vi "validate line configuration.vi"(7 "module":refnum<class "Scan Engine configuration.lvclass">, 11 "Mappings in":T1) -> (1 "valid?":bool, 2 "errors":string, 3 "Mappings out":T1)   [LabVIEW 2013, in "Scan Engine editor node.lvclass"]
uses:
  Scan Engine editor node.lvclass
  Mappings.ctl
  <vilib>/NI/Tag Bus Module Framework/channel/TBM channel.lvclass
  module/configuration/Line.ctl
  Map.ctl
  module/configuration/Scan Engine configuration.lvclass
  <vilib>/NI/Tag Bus/tag/tag descriptor.lvclass/tag descriptor.ctl
  <vilib>/NI/Tag Bus/tag/read tag name.vi
panel:
  in  "warn?":bool
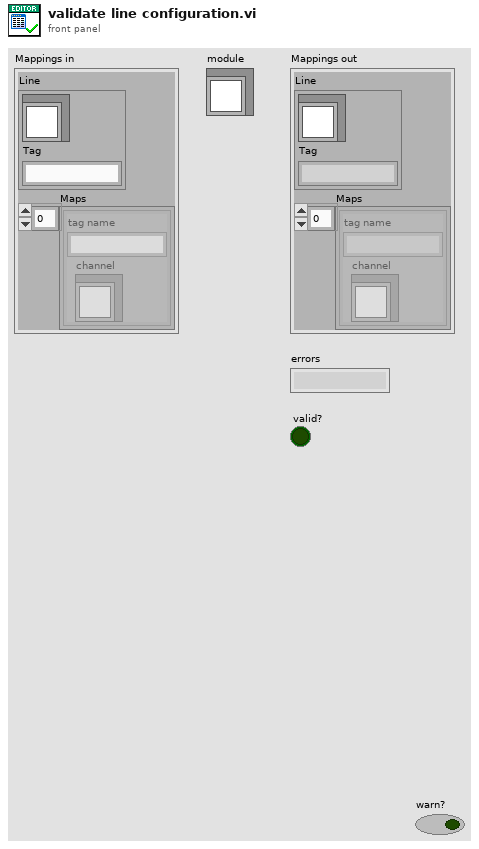
[diagram p1: front panel]
types:
  T1 = typedef "Scan Engine editor node.lvclass/Mappings.ctl" = cluster{"Line":T2, "Maps":T3[]}
  T2 = typedef "Scan Engine configuration.lvclass/Line.ctl" = cluster{"channel":refnum<class "TBM channel.lvclass">, "Tag":string}
  T3 = typedef "Scan Engine editor node.lvclass/Map.ctl" = cluster{"channel":refnum<class "TBM channel.lvclass">, "tag name":string}
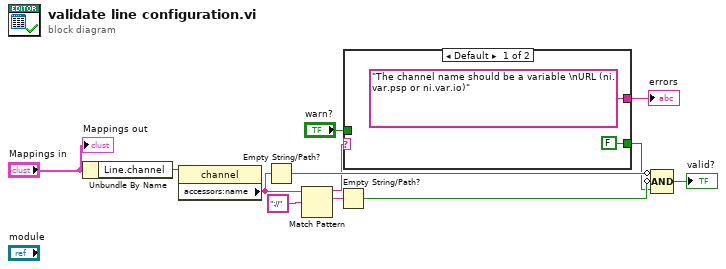
[diagram p0: block diagram]
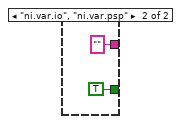
[diagram p2: hidden frame]
diagram:
  n1 = Unbundle By Name("Mappings in") -> ("Line.channel"=w3:refnum<class "TBM channel.lvclass">)
  n2 = property class="channel"(reference=w3) -> ("accessors:name"=w10:string)  [unwired: 1 in, 2 out]
  n3 = Empty String/Path?(string/path=w10) -> (empty?=w11:bool)
  n4 = Match Pattern(string=w10, regular expression="://") -> (before substring=w6:string, match substring=w8:string)  [unwired: 1 in, 2 out]
  n5 = Empty String/Path?(string/path=w8) -> (empty?=w7:bool)
  n6 = case shown="Default" w6 {
    tunnel: [FALSE TRUE] -> w5
    tunnel: "warn?" -> [_ _]
    tunnel: ["The channel name should be a variable \nURL (ni.var.psp or ni.var.io)" ("message") "" ("message")] -> w1
    frame Default {
    }
    frame "ni.var.io", "ni.var.psp" {
    }
  }
  "errors" <- w1
  n7 = Compound Arithmetic op=AND(invert w11, invert w7, w5) -> (→"valid?":bool)
  "Mappings out" <- "Mappings in"
